vi "Untitled 1.vi"() -> ()   [LabVIEW 2019]
uses:
  <vilib>/Instr/_visa.llb/VISA Configure Serial Port (Instr).vi
panel:
  in  "timeout (10sec)":u32=10000
  out "error out":errorcluster
  out "VISA resource name out":refnum<visa-resource-name>
  in  "write buffer":string
  in  "baud rate":u32=9600
  in  "?":bool
  out "Waveform Graph 2":dbl[](graph)
  out "Waveform Graph":dbl[](graph)
  out "Numeric":dbl
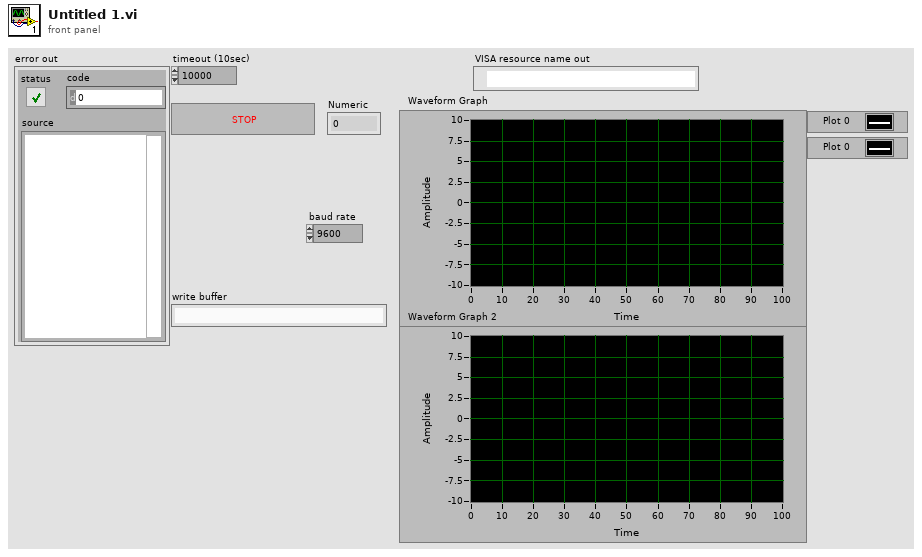
[diagram p1: front panel]
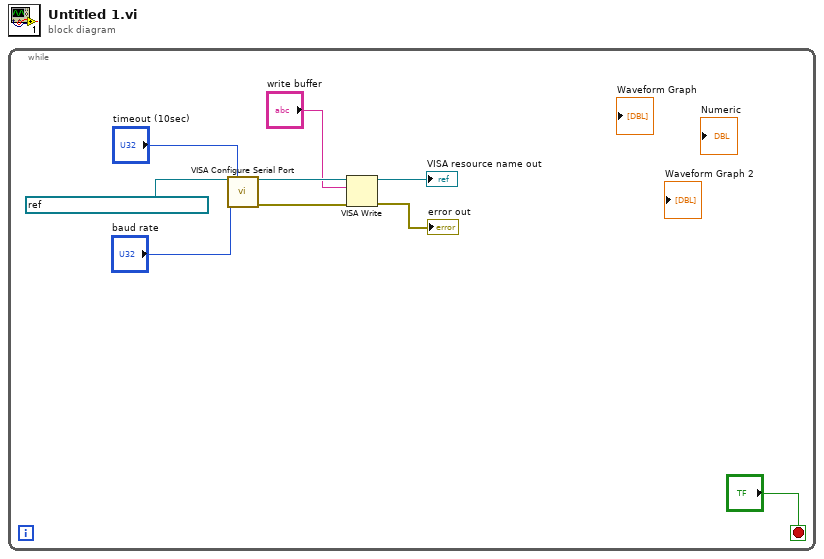
[diagram p0: block diagram]
diagram:
  n1 = while {
    stop <- "?" stop-if-true
    n2 = call-poly "VISA Configure Serial Port"("VISA resource name"=refnum<visa-resource-name> "/dev/cu.usbserial-NX3U1Y58" ("SeialPort Number"), "timeout (10sec)"="timeout (10sec)", "baud rate (9600)"="baud rate") -> ("VISA resource name out"=w7:refnum<visa-resource-name>, "error out"=w5:errorcluster)  [unwired: 11 in]
    n3 = VISA Write(VISA resource name=w7, write buffer="write buffer", error in (no error)=w5) -> (VISA resource name out=→"VISA resource name out":refnum<visa-resource-name>, error out=→"error out":errorcluster)  [unwired: 1 out]
  }
